vi "sine and cos waves controllable by its speed and time.vi"() -> ()   [LabVIEW 2020]
panel:
  in  "Time Target (s)":dbl=1.0
  in  "Slide":dbl(slide) scale=1.0..10.0
  out "Waveform Chart":cluster{dbl, dbl, dbl}(graph)
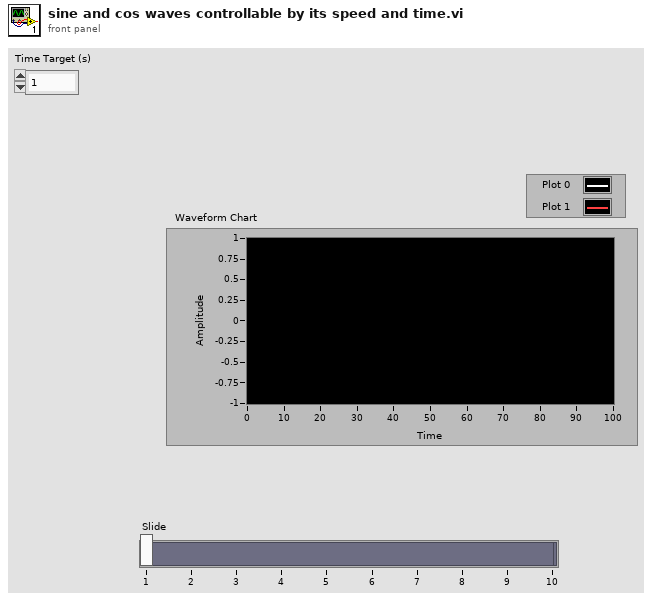
[diagram p1: front panel]
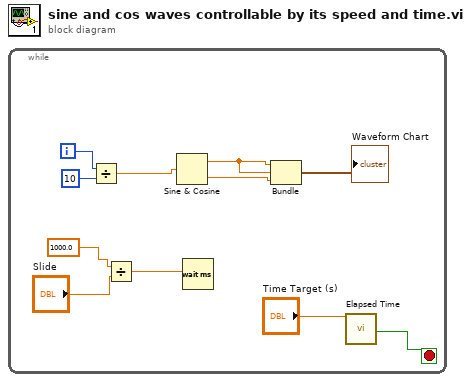
[diagram p0: block diagram]
diagram:
  n1 = while {
    i -> [w11]
    stop <- w4 stop-if-true
    n2 = Divide(x=w11, y=10) -> (x/y=w9:dbl)
    n3 = Divide(x=1000.0 ("y"), y="Slide") -> (x/y=w7:dbl)
    n4 = Sine & Cosine(0:w9) -> (1:w2:dbl, 2:w1:dbl)
    n5 = Wait (ms)(milliseconds to wait=w7) -> ()  [unwired: 1 out]
    n6 = Bundle(w2, w2, w1) -> (→"Waveform Chart":cluster{dbl, dbl, dbl})  [unwired: 1 in]
    n7 = call "Elapsed Time"("Time Target (s)"="Time Target (s)") -> ("Time has Elapsed"=w4:bool)  [unwired: 11 in, 7 out]
  }
